vi "Particle API Example.vi"() -> ()   [LabVIEW 2013]
doc: "Simple example VI that uses the some of the Spark API to interact with a connected Spark device."
uses:
  Controls/Particle Reference.ctl
  <vilib>/httpClient/ClientHandle.ctl
  Controls/Device Query JSON.ctl
  Controls/Devices Query JSON.ctl
  Controls/Function Response JSON.ctl
  Particle API.lvlib
  <vilib>/httpClient/LabVIEWHTTPClient.lvlib
panel:
  out "D7 Function \nResponse":T1
  in  "Blink LED":bool
  out "A0 Function \nResponse":T1
  in  "stop":bool
  in  "Read A0":bool
  in  "Flash Tinker (Mac only)":bool
  in  "Get Current Spark Info":bool
  in  "Login to Spark Account":bool
  out "All Registered Spark Devices":T2=[{"id"="", "name"="", "connected"=TRUE}]
  in  "Spark Password":string
  in  "Spark Username":string
  out "error out":errorcluster
  out "Current Spark Reference Out":T3
  # "Run this VI and select the \"Login to Spark Account\" button, before choosing the other options."
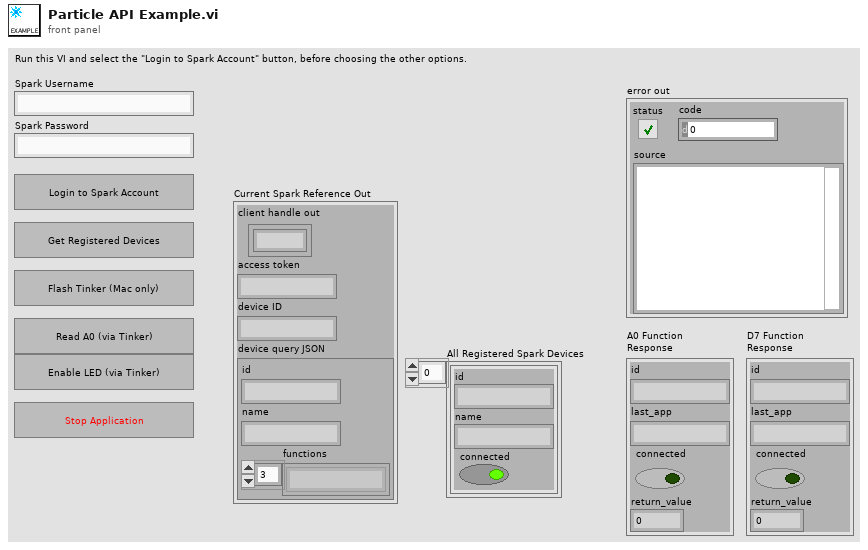
[diagram p1: front panel]
types:
  T1 = typedef "Particle API.lvlib/Function Response JSON.ctl" = cluster{"id":string, "last_app":string, "connected":bool, "return_value":dbl}
  T2 = typedef "Particle API.lvlib/Devices Query JSON.ctl" = cluster{"id":string, "name":string, "connected":bool}[]
  T3 = typedef "Particle API.lvlib/Particle Reference.ctl" = cluster{"client handle out":T4, "access token":string, "device ID":string, "device query JSON":T5}
  T4 = typedef "LabVIEWHTTPClient.lvlib/ClientHandle.ctl" = refnum<k1>
  T5 = typedef "Particle API.lvlib/Device Query JSON.ctl" = cluster{"id":string, "name":string, "functions":string[]}
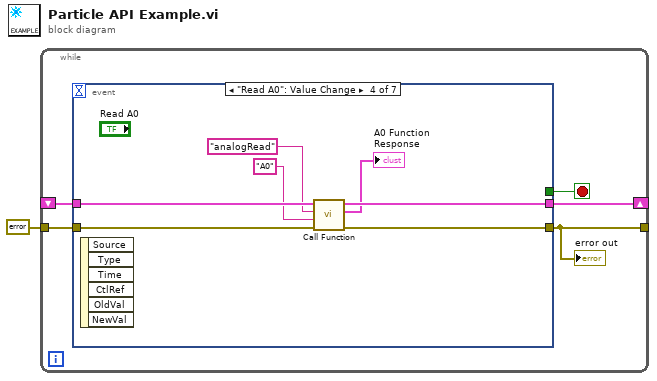
[diagram p0: block diagram]
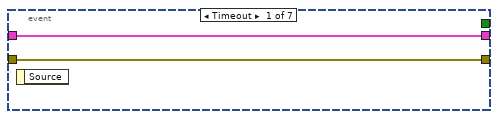
[diagram p2: hidden frame]
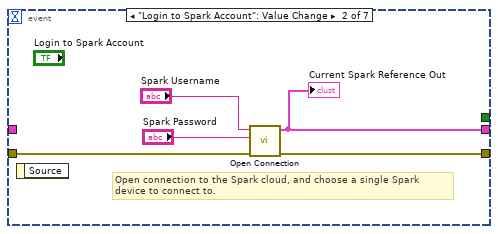
[diagram p3: hidden frame]
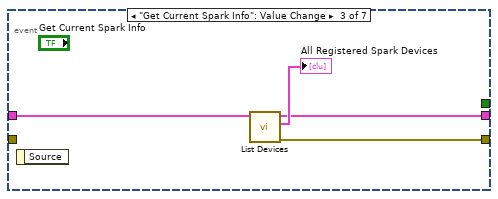
[diagram p4: hidden frame]
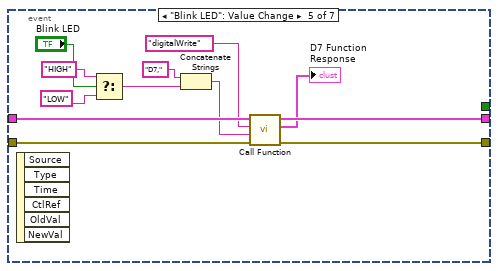
[diagram p5: hidden frame]
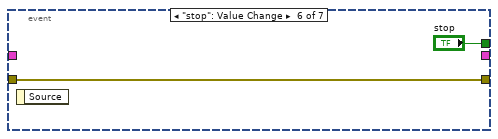
[diagram p6: hidden frame]
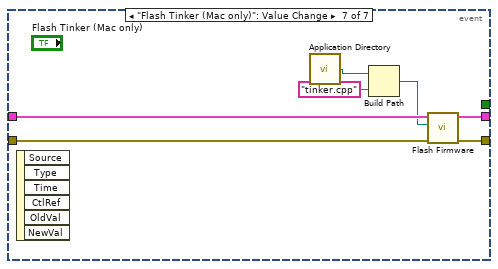
[diagram p7: hidden frame]
diagram:
  n1 = while {
    shift-right: [w6] -> _
    shift-left: _ -> [w5]
    tunnel: errorcluster {"status"=FALSE, "code"=0, "source"=""} ("error out") -> [w3]
    tunnel: [w4] -> _
    stop <- w2 stop-if-true
    n2 = event shown="[3] \"Read A0\": Value Change" {
      selector: _ -> [_ _ _ _ _ _ _]
      dyn-events: _ -> [_ _ _ _ _ _ _]
      timeout: _ -> [_ _ _ _ _ _ _]
      tunnel: [w7 w11 w15 w21 w33 _ w42] -> w6
      tunnel: w5 -> [w7 _ w16 w24 w36 _ w45]
      tunnel: [w8 w10 w14 w22 w34 w38 w43] -> w4
      tunnel: w3 -> [w8 w9 _ w23 w35 w38 w44]
      tunnel: [_ _ _ _ _ "stop" _] -> w2
      event Timeout {
        n3 = event-data() -> ()  [unwired: 1 in, 1 out]
      }
      event "Login to Spark Account": Value Change {
        # "Open connection to the Spark cloud, and choose a single Spark\ndevice to connect to."
        n4 = event-data() -> ()  [unwired: 1 in, 1 out]
        n5 = call "Open Connection.vi"("error in"=w9, "password"="Spark Password", "username"="Spark Username") -> ("error out"=w10:errorcluster, "particle reference out"=w11:T3)  [unwired: 7 in]
        "Current Spark Reference Out" <- w11
      }
      event "Get Current Spark Info": Value Change {
        n6 = event-data() -> ()  [unwired: 1 in, 1 out]
        n7 = call "List Devices.vi"("particle reference in"=w16) -> ("error out"=w14:errorcluster, "devices JSON"=→"All Registered Spark Devices":T2, "particle reference out"=w15:T3)  [unwired: 8 in]
      }
      event "Read A0": Value Change {
        n8 = event-data() -> ()  [unwired: 1 in, 6 out]
        n9 = call "Call Function.vi"("error in"=w23, "arguments"="A0" ("Arguments"), "function name"="analogRead" ("Function Name"), "particle reference in"=w24) -> ("error out"=w22:errorcluster, "function response"=→"A0 Function \nResponse":T1, "particle reference out"=w21:T3)  [unwired: 5 in]
      }
      event "Blink LED": Value Change {
        n10 = event-data() -> ()  [unwired: 1 in, 6 out]
        n11 = Select(t="HIGH", s="Blink LED", f="LOW") -> (s? t:f=w25:string)
        n12 = Concatenate Strings("D7," ("Arguments"), w25) -> (w26:string)
        n13 = call "Call Function.vi"("error in"=w35, "arguments"=w26, "function name"="digitalWrite" ("Function Name"), "particle reference in"=w36) -> ("error out"=w34:errorcluster, "function response"=→"D7 Function \nResponse":T1, "particle reference out"=w33:T3)  [unwired: 5 in]
      }
      event "stop": Value Change {
        n14 = event-data() -> ()  [unwired: 1 in, 1 out]
      }
      event "Flash Tinker (Mac only)": Value Change {
        n15 = event-data() -> ()  [unwired: 1 in, 6 out]
        n16 = call <vilib>:"Application Directory.vi"() -> ("Application Directory"=w41:path)
        n17 = Build Path(base path=w41, name or relative path="tinker.cpp") -> (appended path=w39:path)
        n18 = call "Flash Firmware.vi"("error in"=w44, "path to code"=w39, "particle reference in"=w45) -> ("error out"=w43:errorcluster, "particle reference out"=w42:T3)  [unwired: 7 in]
      }
    }
    "error out" <- w4
  }
